vi "Get Position.vi"(8 "error in (no error)":errorcluster) -> (0 "error out":errorcluster, 1 "Z Pos":dbl[](array[numeric]), 2 "Y Pos":dbl[](array[numeric]), 3 "X Pos":dbl[](array[numeric]))   [LabVIEW 2011]
panel:
  in  "VISA resource name":refnum<visa-resource-name>
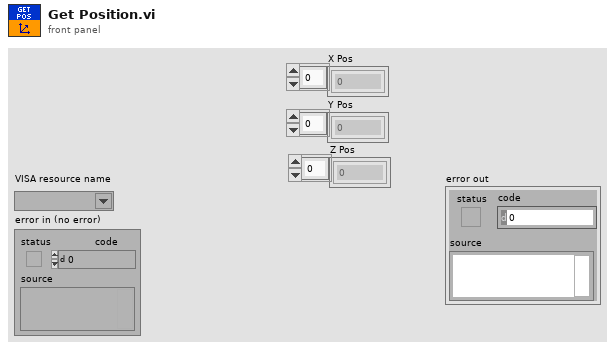
[diagram p1: front panel]
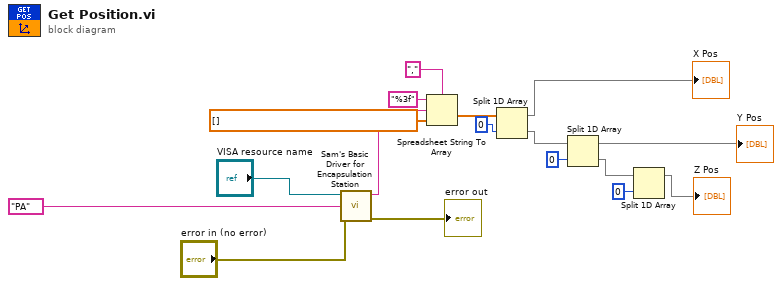
[diagram p0: block diagram]
diagram:
  n1 = call "Sam's Basic Driver for Encapsulation Station.vi"("error in (no error)"="error in (no error)", "Combo Box"="PA", "VISA resource name"="VISA resource name") -> ("error out"=→"error out":errorcluster, "read buffer 2"=w12:string)  [unwired: 6 in, 1 out]
  n2 = Spreadsheet String To Array(delimiter (Tab)=",", format string="%3f", spreadsheet string=w12, array type (2D Dbl)=dbl[] []) -> (array=w10:dbl[])
  n3 = Split 1D Array(array=w10, index=0 ("index (row)")) -> (first subarray=→"X Pos":dbl[], second subarray=w6:dbl[])
  n4 = Split 1D Array(array=w6, index=0) -> (first subarray=→"Y Pos":dbl[], second subarray=w4:dbl[])
  n5 = Split 1D Array(array=w4, index=0) -> (first subarray=→"Z Pos":dbl[])  [unwired: 1 out]
